vi "OnOff.vi"(0 "setpoint off":dbl step=0.01 format="%.2f", 1 "X1(SetState)":i32, 5 "setpoint on":dbl step=0.01 format="%.2f", 7 "process variable":dbl step=0.01 format="%.2f", 9 "manual control":bool) -> (4 "output":bool)   [LabVIEW 2019, in "control.lvlib"]
uses:
  control.lvlib
  Trigers/Triggers.lvlib
panel:
  # "Входы\nX1(SetState) заданное состояние\n     0 – аварийное значение\n     1 – минимум\n     2 – стоп\n     3 – ручной\n     4 – автомат\n     5 – максимум"
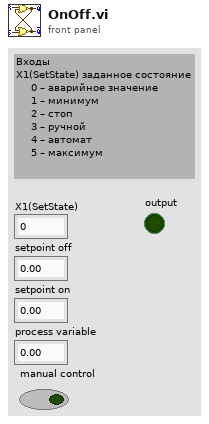
[diagram p1: front panel]
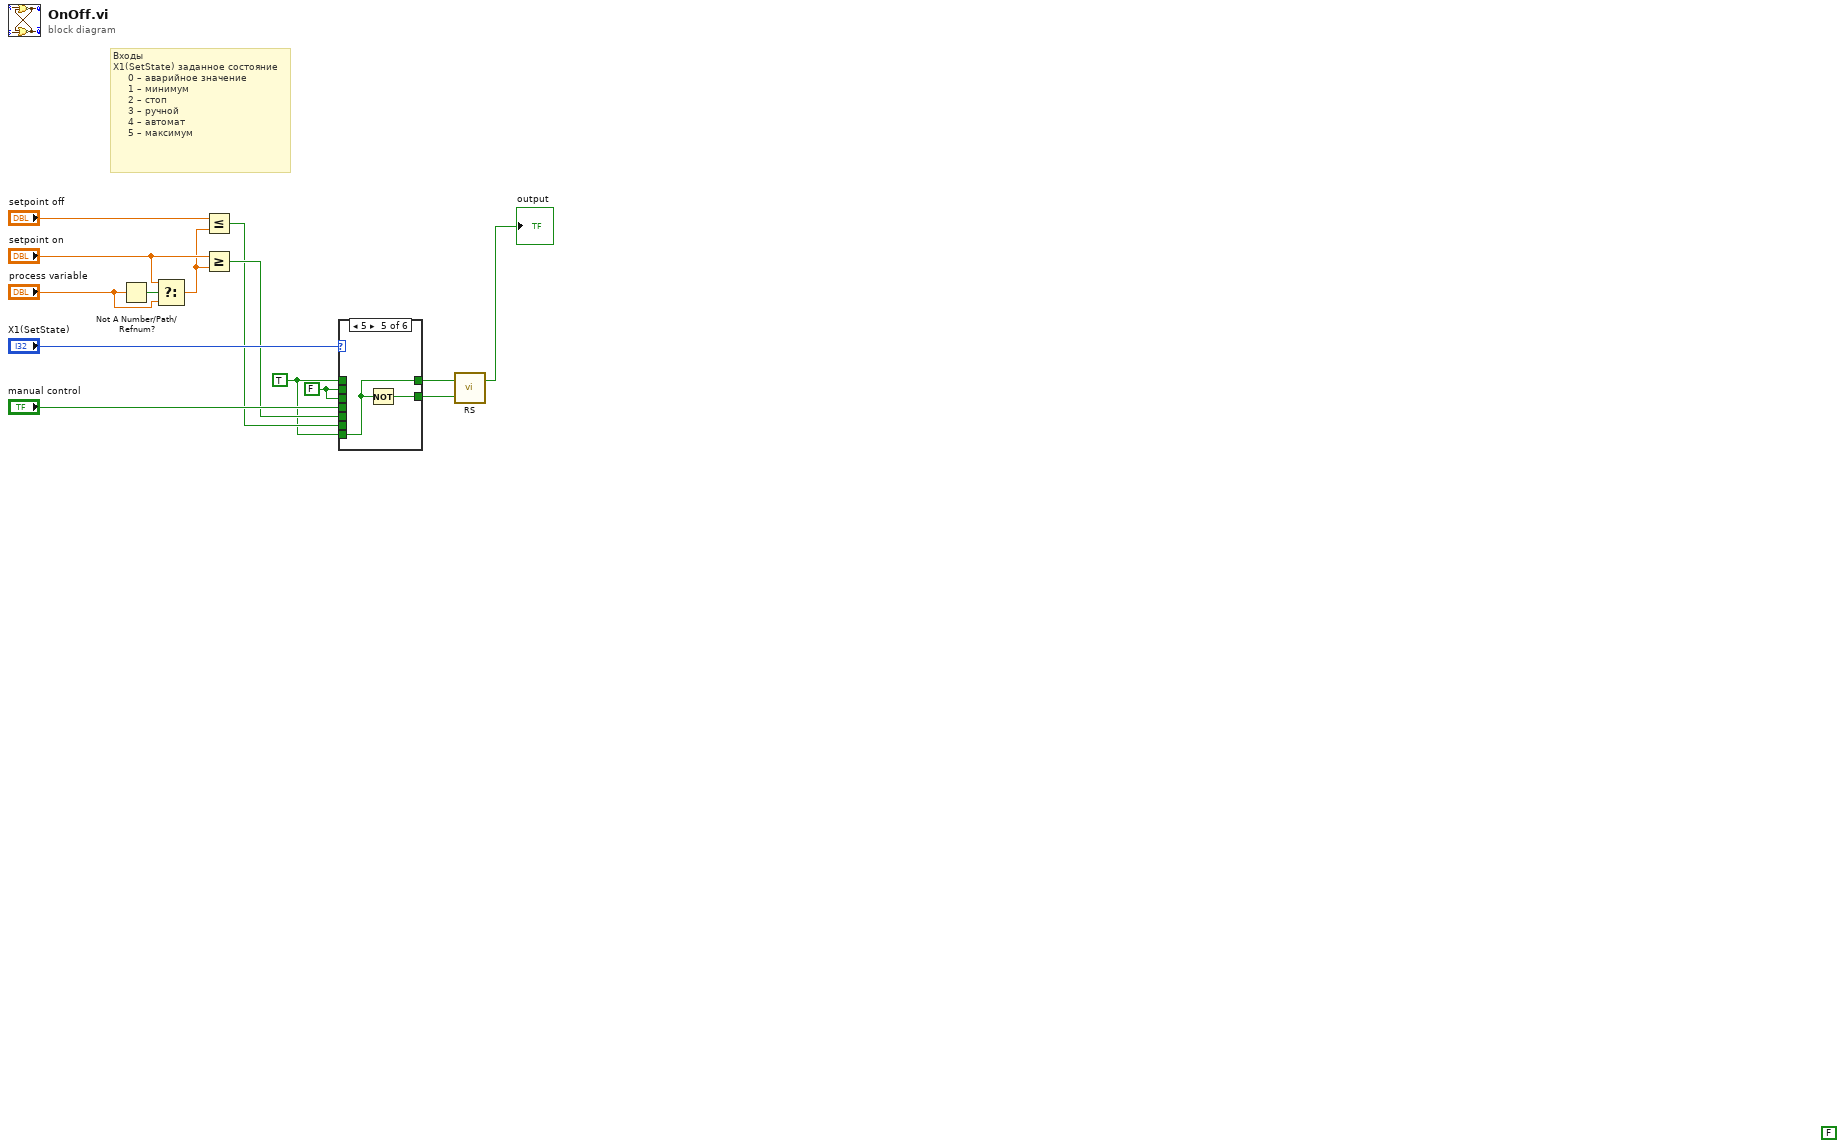
[diagram p0: block diagram]
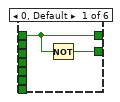
[diagram p2: hidden frame]
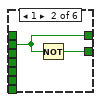
[diagram p3: hidden frame]
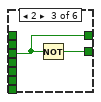
[diagram p4: hidden frame]
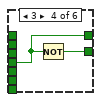
[diagram p5: hidden frame]
diagram:
  w2 = TRUE
  w7 = FALSE
  (unwired) FALSE
  # "Входы\nX1(SetState) заданное состояние\n     0 – аварийное значение\n     1 – минимум\n     2 – стоп\n     3 – ручной\n     4 – автомат\n     5 – максимум"
  n1 = Not A Number/Path/Refnum?(number/path/refnum="process variable") -> (NaN/Path/Refnum?=w9:bool)
  n2 = Select(t="setpoint on", s=w9, f="process variable") -> (s? t:f=w8:dbl)
  n3 = Less Or Equal?(x="setpoint off", y=w8) -> (x <= y?=w5:bool)
  n4 = Greater Or Equal?(x="setpoint on", y=w8) -> (x >= y?=w6:bool)
  n5 = case shown="5" "X1(SetState)" {
    tunnel: w7 -> [_ w17 _ _ _ _]
    tunnel: w2 -> [_ _ _ _ w23 _]
    tunnel: [w16 w17 w19 w21 w23 w26] -> w3
    tunnel: w2 -> [w16 _ _ _ _ _]
    tunnel: "manual control" -> [_ _ _ w21 _ _]
    tunnel: w7 -> [_ _ w19 _ _ _]
    tunnel: w6 -> [_ _ _ _ _ w26]
    tunnel: w5 -> [_ _ _ _ _ w25]
    tunnel: [w15 w18 w20 w22 w24 w25] -> w4
    frame 0, Default {
      n6 = Not(x=w16) -> (.not. x?=w15:bool)
    }
    frame 1 {
      n7 = Not(x=w17) -> (.not. x?=w18:bool)
    }
    frame 2 {
      n8 = Not(x=w19) -> (.not. x?=w20:bool)
    }
    frame 3 {
      n9 = Not(x=w21) -> (.not. x?=w22:bool)
    }
    frame 5 {
      n10 = Not(x=w23) -> (.not. x?=w24:bool)
    }
    frame 4 {
    }
  }
  n11 = call "RS.vi"("R"=w4, "S"=w3) -> ("Q"=→"output":bool)  [unwired: 1 out]
